vi "subscribe.vi"   [LabVIEW 2023, in "Publisher Subscriber.lvlib"]
uses:
  <userlib>/_Publisher Subscriber/Publisher Subscriber.lvlib
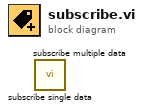
[diagram p0: block diagram]
diagram:
  n1 = call <userlib>:"subscribe single data.vi"() -> ()  [unwired: 10 in, 2 out]
  n2 = call <userlib>:"subscribe multiple data.vi"() -> ()  [unwired: 10 in, 2 out]
